vi "Numeric GTLT.vi"(11 "Data In":i32) -> (3 "Data Out":i32)   [LabVIEW 2016]
uses:
  Core/Assert API Components/Failure Actions.ctl
  Core/Assert API Components/Assert API Components.lvlib
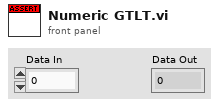
[diagram p1: front panel]
types:
  T1 = typedef "Assert API Components.lvlib/Failure Actions.ctl" = enum16{"None", "Log To File", "Pause Execution", "Abort Execution"}
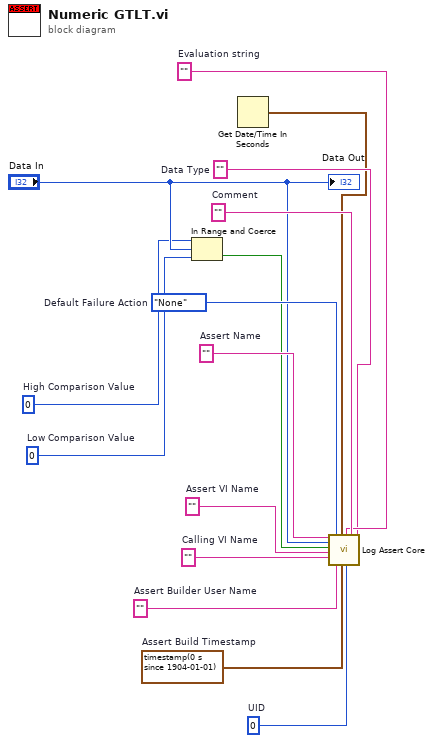
[diagram p0: block diagram]
diagram:
  w1 = 0  # UID
  w3 = ""  # Assert VI Name
  w4 = ""  # Calling VI Name
  w5 = ""  # Assert Builder User Name
  w6 = timestamp(0 s since 1904-01-01)  # Assert Build Timestamp
  w7 = ""  # Data Type
  w10 = 0  # High Comparison Value
  w12 = ""  # Comment
  w8 = ""  # Evaluation string
  w14 = Failure_Actions."None"  # Default Failure Action
  w15 = ""  # Assert Name
  w13 = 0  # Low Comparison Value
  n1 = In Range and Coerce(upper limit=w10, x="Data In", lower limit=w13) -> (In Range?=w9:bool)  [unwired: 1 out]
  n2 = Get Date/Time In Seconds() -> (seconds since 1Jan1904=w2:timestamp)
  n3 = call "Log Assert Core.vi"("Assert Name"=w15, "Data Value"="Data In", "Status"=w9, "Assert VI Name"=w3, "Calling VI Name"=w4, "Failure Action"=w14, "Assert Builder User Name"=w5, "Last Update"=w2, "Assert Build Timestamp"=w6, "Evaluation String"=w8, "Assert VI UID"=w1, "Comment"=w12, "Data Type"=w7) -> ()  [unwired: 7 in]
  "Data Out" <- "Data In"
